vi "Populate Objects List.vi"(8 "error in":errorcluster, 11 "UI Actor in":refnum<class "UI Actor.lvclass">) -> (0 "error out":errorcluster, 3 "UI Actor out":refnum<class "UI Actor.lvclass">)   [LabVIEW 2024, in "UI Actor.lvlib" / "UI Actor.lvclass"]
uses:
  UI Actor.lvclass
  UI Actor.lvclass/UI Actor.ctl
  Core/EDS/EDS.lvclass
  Core/Mandatory Objects/Mandatory Objects.lvclass
panel:
  out "Mandatory Objects":refnum<class "Mandatory Objects.lvclass">
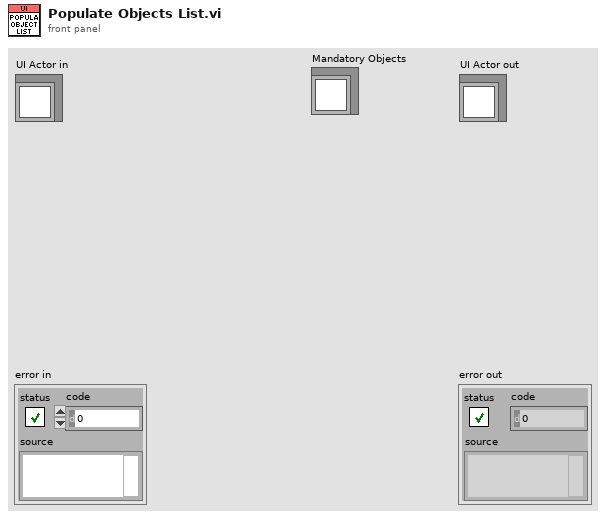
[diagram p1: front panel]
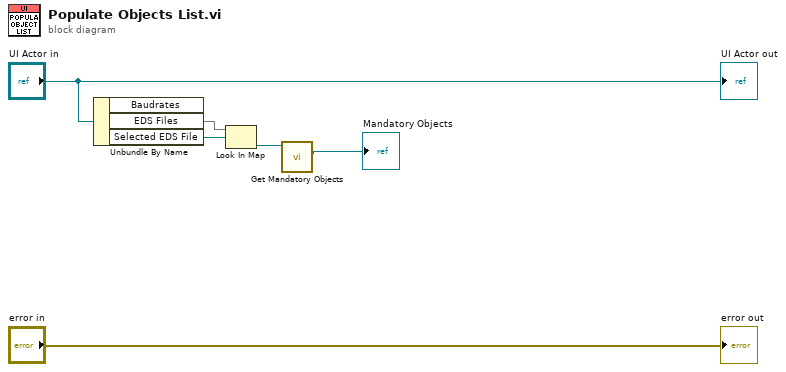
[diagram p0: block diagram]
diagram:
  n1 = Unbundle By Name("UI Actor in") -> ("EDS Files"=w5:map{path, refnum<class "EDS.lvclass">}, "Selected EDS File"=w4:path)  [unwired: 1 out]
  n2 = Look In Map(map=w5, key=w4) -> (value=w2:refnum<class "EDS.lvclass">)  [unwired: 1 in, 1 out]
  n3 = call "Get Mandatory Objects.vi"("EDS in"=w2) -> ("Mandatory Objects"=→"Mandatory Objects":refnum<class "Mandatory Objects.lvclass">)  [unwired: 9 in, 1 out]
  "error out" <- "error in"
  "UI Actor out" <- "UI Actor in"
